vi "GetBinlogdllpath.vi"() -> (3 "dup path":path)   [LabVIEW 2015, in "Read Write BLF.lvclass"]
uses:
  BLF/Read Write BLF.lvclass
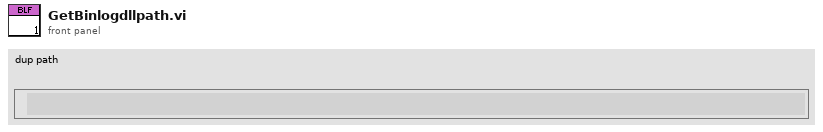
[diagram p1: front panel]
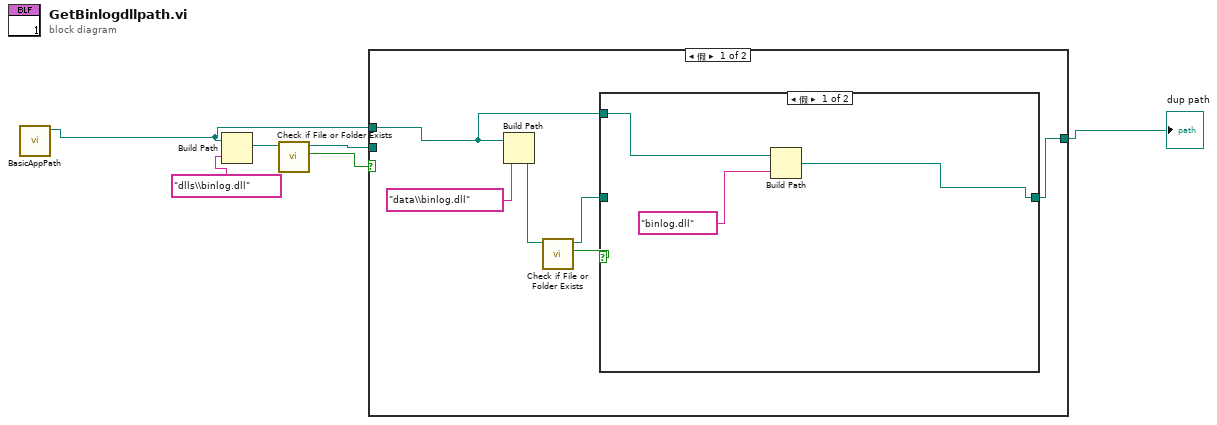
[diagram p0: block diagram]
diagram:
  n1 = call "BasicAppPath.vi"() -> ("AppPath"=w1:path)  [unwired: 10 in, 1 out]
  n2 = Build Path(base path=w1, name or relative path="dlls\\binlog.dll" ("名称或相对路径")) -> (appended path=w5:path)
  n3 = call <vilib>:"Check if File or Folder Exists.vi"("path"=w5) -> ("file or folder exists?"=w4:bool, "dup path"=w3:path)  [unwired: 8 in, 1 out]
  n4 = case shown="假" w4 {
    tunnel: w3 -> [_ w17]
    tunnel: [w8 w17] -> w2
    tunnel: w1 -> [w7 _]
    frame False {
      n5 = Build Path(base path=w7, name or relative path="data\\binlog.dll" ("名称或相对路径")) -> (appended path=w11:path)
      n6 = call <vilib>:"Check if File or Folder Exists.vi"("path"=w11) -> ("file or folder exists?"=w10:bool, "dup path"=w9:path)  [unwired: 8 in, 1 out]
      n7 = case shown="假" w10 {
        tunnel: w9 -> [_ w16]
        tunnel: [w13 w16] -> w8
        tunnel: w7 -> [w15 _]
        frame False {
          n8 = Build Path(base path=w15, name or relative path="binlog.dll" ("名称或相对路径")) -> (appended path=w13:path)
        }
        frame True {
        }
      }
    }
    frame True {
    }
  }
  "dup path" <- w2
